vi "Calculate - Controller.vi"() -> ()   [LabVIEW 2013]
uses:
  Controller/Controller.lvclass
  <vilib>/ActorFramework/Message Queue/Message Queue.lvclass/Message Queue.ctl
  Controller Messages/Execute Operation Msg/Execute Operation Msg.lvclass/Execute Operation Msg.ctl
  <vilib>/ActorFramework/Message Enqueuer/Message Enqueuer.lvclass/Message Enqueuer.ctl
  Controller Messages/Get Operation Results Msg/Get Operation Results Msg.lvclass/Get Operation Results Msg.ctl
  <vilib>/ActorFramework/Stop Msg/Stop Msg.lvclass/Stop Msg.ctl
  <vilib>/ActorFramework/Message Enqueuer/Enqueue.vi
  <vilib>/ActorFramework/Message Enqueuer/Enqueue Critical.vi
  <vilib>/ActorFramework/Message Priority Queue/Priority Enqueue.vi
  Simulation/Simulation Data_Global.vi
  Controller Messages/Execute Operation Msg/Execute Operation Msg.lvclass
  Controller Messages/Get Operation Results Msg/Get Operation Results Msg.lvclass
  <vilib>/ActorFramework/Stop Msg/Stop Msg.lvclass
  <vilib>/ActorFramework/Actor/Actor.lvclass
  <vilib>/ActorFramework/Message Queue/Message Queue.lvclass
  Simulation/Simulation.lvlib
panel:
  in  "btnDivide":bool
  in  "btnMultiply":bool
  in  "btnSubtract":bool
  in  "btnStop":bool
  in  "btnAdd":bool
  out "Result":dbl
  in  "Operand 2":dbl
  in  "Operand 1":dbl
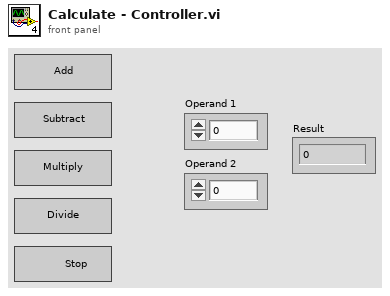
[diagram p1: front panel]
types:
  T1 = enum16{"Addition", "Subtraction", "Multiply", "Divide"}
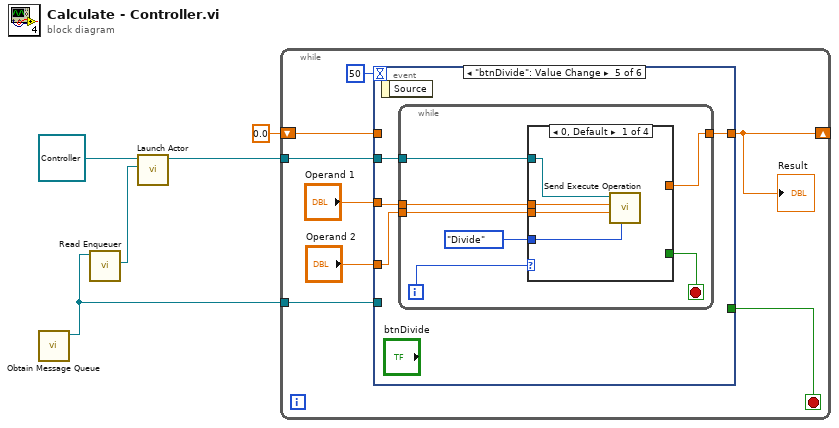
[diagram p0: block diagram]
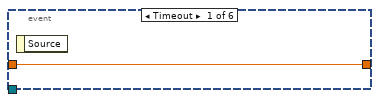
[diagram p2: hidden frame]
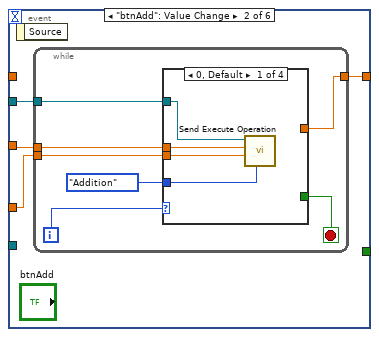
[diagram p3: hidden frame]
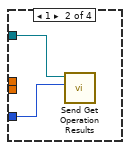
[diagram p4: hidden frame]
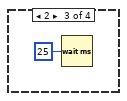
[diagram p5: hidden frame]
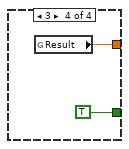
[diagram p6: hidden frame]
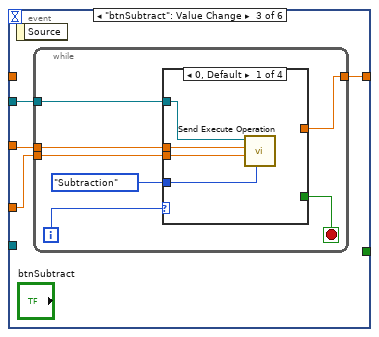
[diagram p7: hidden frame]
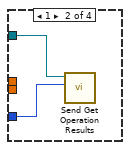
[diagram p8: hidden frame]
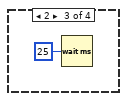
[diagram p9: hidden frame]
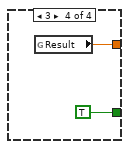
[diagram p10: hidden frame]
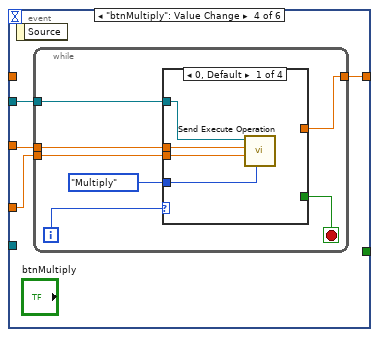
[diagram p11: hidden frame]
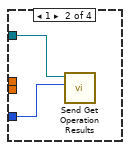
[diagram p12: hidden frame]
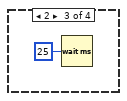
[diagram p13: hidden frame]
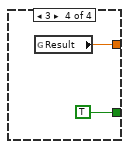
[diagram p14: hidden frame]
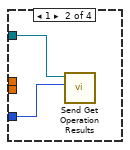
[diagram p15: hidden frame]
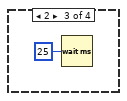
[diagram p16: hidden frame]
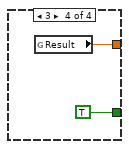
[diagram p17: hidden frame]
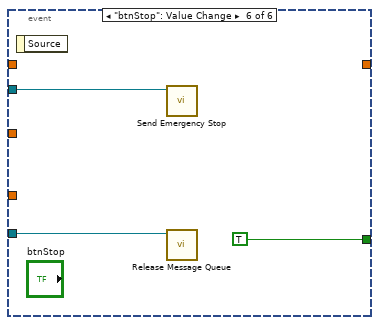
[diagram p18: hidden frame]
diagram:
  n1 = call <vilib>:"Obtain Message Queue.vi"() -> ("Message Queue"=w2:refnum<class "Message Queue.lvclass">)  [unwired: 10 in, 1 out]
  n2 = call <vilib>:"Read Enqueuer.vi"("Message Queue"=w2) -> ("Message Enqueuer"=w4:refnum<class "Message Enqueuer.lvclass">)  [unwired: 10 in]
  n3 = call <vilib>:"Launch Actor.vi"("Actor-to-Caller Enqueuer"=w4, "Actor"=refnum<class "Controller.lvclass"> refnum ("Controller.lvlib:Controller.lvclass")) -> ("Caller-To-Actor Enqueuer"=w3:refnum<class "Message Enqueuer.lvclass">)  [unwired: 8 in, 1 out]
  n4 = while {
    tunnel: w3 -> [w13]
    tunnel: w2 -> [w12]
    shift-right: [w6] -> _
    shift-left: 0.0 -> [w8]
    stop <- w11 stop-if-true
    n5 = event shown="[4] \"btnDivide\": Value Change" {
      selector: _ -> [_ _ _ _ _ _]
      dyn-events: _ -> [_ _ _ _ _ _]
      timeout: 50 -> [_ _ _ _ _ _]
      tunnel: w13 -> [_ w16 w36 w56 w76 w97]
      tunnel: w12 -> [_ _ _ _ _ w96]
      tunnel: [_ _ _ _ _ TRUE] -> w11
      tunnel: "Operand 1" -> [_ w18 w38 w58 w78 _]
      tunnel: "Operand 2" -> [_ w17 w37 w57 w77 _]
      tunnel: w8 -> [w14 _ _ _ _ _]
      tunnel: [w14 w15 w35 w55 w75 _] -> w6
      event Timeout {
        n6 = event-data() -> ()  [unwired: 1 in, 1 out]
      }
      event "btnAdd": Value Change {
        n7 = event-data() -> ()  [unwired: 1 in, 1 out]
        n8 = while {
          tunnel: w18 -> [w25]
          tunnel: w17 -> [w24]
          tunnel: w16 -> [w23]
          tunnel: [w20] -> w15
          i -> [w22]
          stop <- w19 stop-if-true
          n9 = case shown="0, Default" w22 {
            tunnel: w25 -> [w29 _ _ _]
            tunnel: w24 -> [w28 _ _ _]
            tunnel: w23 -> [w27 w31 _ _]
            tunnel: T1."Addition" ("Operation") -> [w26 w30 _ _]
            tunnel: [_ _ _ w34] -> w20
            tunnel: [_ _ _ TRUE] -> w19
            frame 0, Default {
              n10 = call "Send Execute Operation.vi"("Operation"=w26, "Op 2"=w28, "Op 1"=w29, "Message Enqueuer"=w27) -> ()  [unwired: 6 in, 2 out]
            }
            frame 1 {
              n11 = call "Send Get Operation Results.vi"("Operation"=w30, "Message Enqueuer"=w31) -> ()  [unwired: 8 in, 2 out]
            }
            frame 2 {
              n12 = Wait (ms)(milliseconds to wait=u32 25) -> ()  [unwired: 1 out]
            }
            frame 3 {
              n13 = global read "Simulation Data_Global.vi" "Result"() -> (w34:dbl)
            }
          }
        }
      }
      event "btnSubtract": Value Change {
        n14 = event-data() -> ()  [unwired: 1 in, 1 out]
        n15 = while {
          tunnel: w38 -> [w45]
          tunnel: w37 -> [w44]
          tunnel: w36 -> [w43]
          tunnel: [w40] -> w35
          i -> [w42]
          stop <- w39 stop-if-true
          n16 = case shown="0, Default" w42 {
            tunnel: w45 -> [w49 _ _ _]
            tunnel: w44 -> [w48 _ _ _]
            tunnel: w43 -> [w47 w51 _ _]
            tunnel: T1."Subtraction" ("Operation") -> [w46 w50 _ _]
            tunnel: [_ _ _ w54] -> w40
            tunnel: [_ _ _ TRUE] -> w39
            frame 0, Default {
              n17 = call "Send Execute Operation.vi"("Operation"=w46, "Op 2"=w48, "Op 1"=w49, "Message Enqueuer"=w47) -> ()  [unwired: 6 in, 2 out]
            }
            frame 1 {
              n18 = call "Send Get Operation Results.vi"("Operation"=w50, "Message Enqueuer"=w51) -> ()  [unwired: 8 in, 2 out]
            }
            frame 2 {
              n19 = Wait (ms)(milliseconds to wait=u32 25) -> ()  [unwired: 1 out]
            }
            frame 3 {
              n20 = global read "Simulation Data_Global.vi" "Result"() -> (w54:dbl)
            }
          }
        }
      }
      event "btnMultiply": Value Change {
        n21 = event-data() -> ()  [unwired: 1 in, 1 out]
        n22 = while {
          tunnel: w58 -> [w65]
          tunnel: w57 -> [w64]
          tunnel: w56 -> [w63]
          tunnel: [w60] -> w55
          i -> [w62]
          stop <- w59 stop-if-true
          n23 = case shown="0, Default" w62 {
            tunnel: w65 -> [w69 _ _ _]
            tunnel: w64 -> [w68 _ _ _]
            tunnel: w63 -> [w67 w71 _ _]
            tunnel: T1."Multiply" ("Operation") -> [w66 w70 _ _]
            tunnel: [_ _ _ w74] -> w60
            tunnel: [_ _ _ TRUE] -> w59
            frame 0, Default {
              n24 = call "Send Execute Operation.vi"("Operation"=w66, "Op 2"=w68, "Op 1"=w69, "Message Enqueuer"=w67) -> ()  [unwired: 6 in, 2 out]
            }
            frame 1 {
              n25 = call "Send Get Operation Results.vi"("Operation"=w70, "Message Enqueuer"=w71) -> ()  [unwired: 8 in, 2 out]
            }
            frame 2 {
              n26 = Wait (ms)(milliseconds to wait=u32 25) -> ()  [unwired: 1 out]
            }
            frame 3 {
              n27 = global read "Simulation Data_Global.vi" "Result"() -> (w74:dbl)
            }
          }
        }
      }
      event "btnDivide": Value Change {
        n28 = event-data() -> ()  [unwired: 1 in, 1 out]
        n29 = while {
          tunnel: w78 -> [w85]
          tunnel: w77 -> [w84]
          tunnel: w76 -> [w83]
          tunnel: [w80] -> w75
          i -> [w82]
          stop <- w79 stop-if-true
          n30 = case shown="0, Default" w82 {
            tunnel: w85 -> [w89 _ _ _]
            tunnel: w84 -> [w88 _ _ _]
            tunnel: w83 -> [w87 w91 _ _]
            tunnel: T1."Divide" ("Operation") -> [w86 w90 _ _]
            tunnel: [_ _ _ w94] -> w80
            tunnel: [_ _ _ TRUE] -> w79
            frame 0, Default {
              n31 = call "Send Execute Operation.vi"("Operation"=w86, "Op 2"=w88, "Op 1"=w89, "Message Enqueuer"=w87) -> ()  [unwired: 6 in, 2 out]
            }
            frame 1 {
              n32 = call "Send Get Operation Results.vi"("Operation"=w90, "Message Enqueuer"=w91) -> ()  [unwired: 8 in, 2 out]
            }
            frame 2 {
              n33 = Wait (ms)(milliseconds to wait=u32 25) -> ()  [unwired: 1 out]
            }
            frame 3 {
              n34 = global read "Simulation Data_Global.vi" "Result"() -> (w94:dbl)
            }
          }
        }
      }
      event "btnStop": Value Change {
        n35 = event-data() -> ()  [unwired: 1 in, 1 out]
        n36 = call <vilib>:"Send Emergency Stop.vi"("Message Enqueuer"=w97) -> ()  [unwired: 10 in, 1 out]
        n37 = call <vilib>:"Release Message Queue.vi"("Message Queue"=w96) -> ()  [unwired: 9 in, 2 out]
      }
    }
    "Result" <- w6
  }
